vi "DetectExtendCollision.vi"(4 "Ball":T1, 5 "Goal":dbl[](array[numeric]), 6 "Robot in":T2={"id"=0, "function"=enum."Attacker", "x"=0.0, "y"=0.0, "orientation"=0.0, "v_tangent"=0.0, "v_normal"=0.0, "v_ang"=0.0, "kick_x"=0.0, "kick_z"=0.0, "dribble"=FALSE, "Timestamp"=timestamp(0 s since 1904-01-01), "estimatives"={"est_v_tangent"=0.0, "est_v_normal"=0.0, "est_vx"=0.0, "est_vy"=0.0, "Pos Robot Est"=[]}, "dest_x_kick"=0.0, "dest_y_kick"=0.0, "Gap Coord"=[], "States"=enum."GoToTangent", "Path "=[], "Path  Smooth"=[], "Dest"=[]}, 7 "Initial State":dbl[](array[numeric]), 9 "enemy_robots":T2[](array[typedef]), 10 "Point":dbl[](array[numeric]), 11 "our_robots":T2[](array[typedef])) -> (2 "Collision":bool)   [LabVIEW 2017]
uses:
  Core/AI Robot.ctl
  Intel/Functions Enum.ctl
  Intel/AttackerStates.ctl
  PathDests.ctl
  PathDest.ctl
  Core/AI Ball.ctl
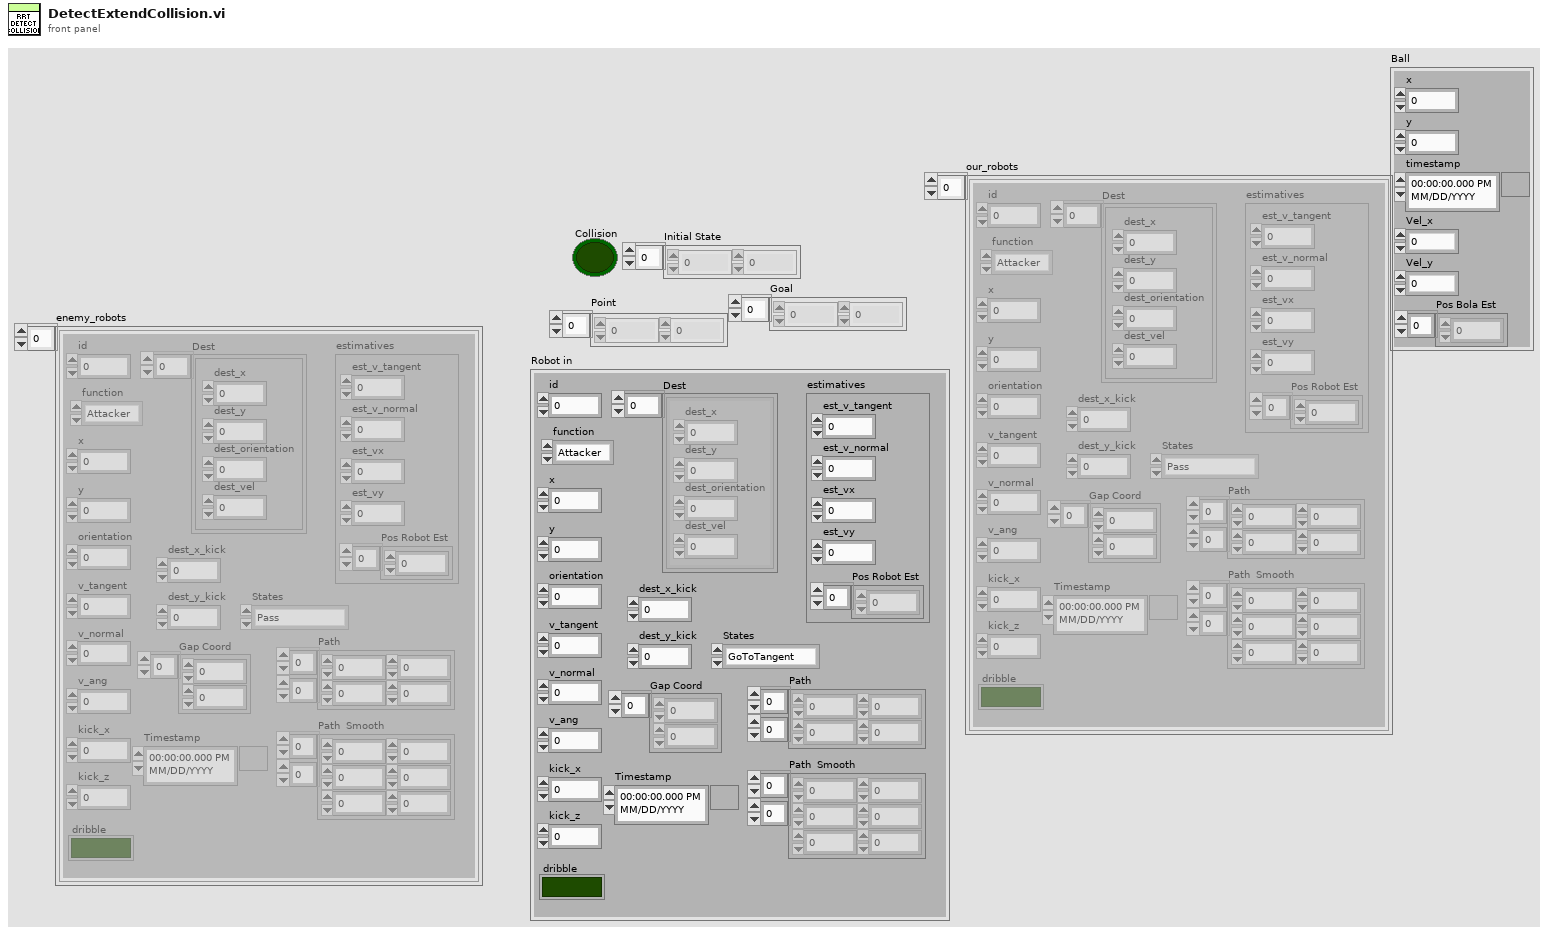
[diagram p1: front panel]
types:
  T1 = typedef "AI Ball.ctl" = cluster{"x":dbl, "y":dbl, "timestamp":timestamp, "Vel_x":dbl, "Vel_y":dbl, "Pos Bola Est":dbl[]}
  T2 = typedef "AI Robot.ctl" = cluster{"id":u32, "function":T3, "x":dbl, "y":dbl, "orientation":dbl, "v_tangent":dbl, "v_normal":dbl, "v_ang":dbl, "kick_x":dbl, "kick_z":dbl, "dribble":bool, "Timestamp":timestamp, "estimatives":cluster{"est_v_tangent":dbl, "est_v_normal":dbl, "est_vx":dbl, "est_vy":dbl, "Pos Robot Est":dbl[]}, "dest_x_kick":dbl, "dest_y_kick":dbl, "Gap Coord":dbl[], "States":T4, "Path ":dbl[][], "Path  Smooth":dbl[][], "Dest":T5}
  T3 = typedef "Functions Enum.ctl" = enum16{"Attacker", "Goalie", "Defender", "Striker", "Goto 0", "Dummy", "Kicker", "ZigZag"}
  T4 = typedef "AttackerStates.ctl" = enum16{"Pass", "GoToTangent", "BallGetting", "GoToKick", ""}
  T5 = typedef "PathDests.ctl" = T6[]
  T6 = typedef "PathDest.ctl" = cluster{"dest_x":dbl, "dest_y":dbl, "dest_orientation":dbl, "dest_vel":dbl}
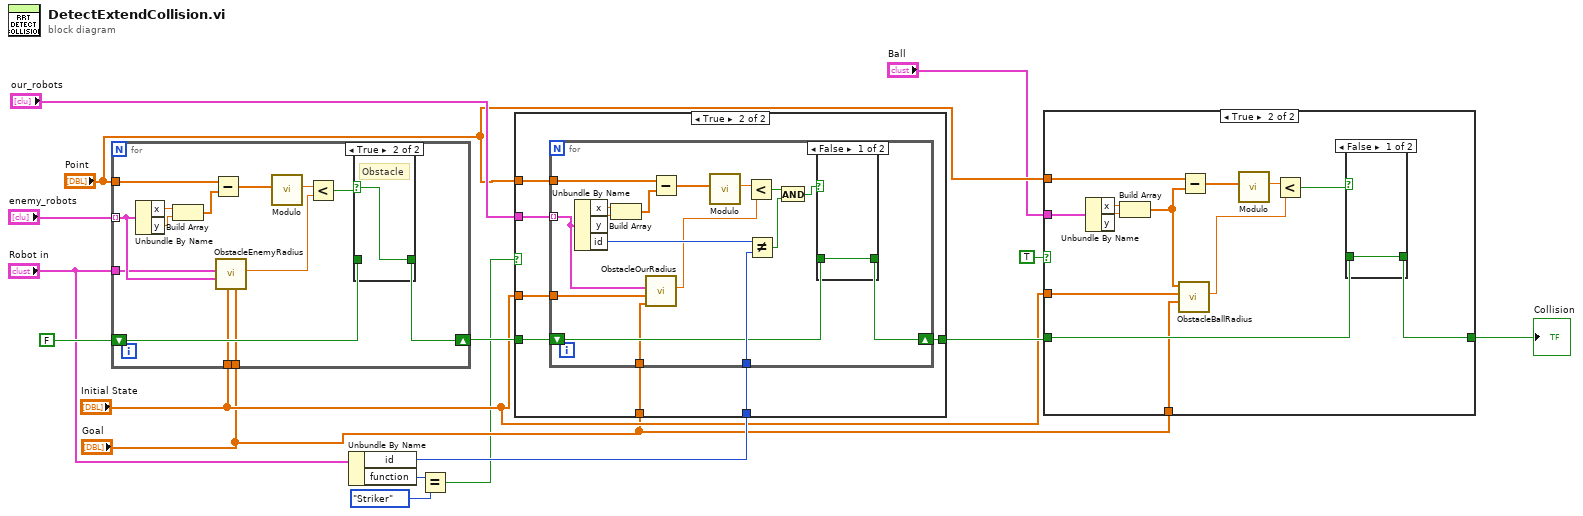
[diagram p0: block diagram]
diagram:
  n1 = for {
    tunnel: "enemy_robots" -> [w20] mode=indexing
    tunnel: "Point" -> [w27]
    shift-right: [w22] -> w11
    shift-left: FALSE -> [w23]
    tunnel: "Robot in" -> [w19]
    tunnel: "Initial State" -> [w18]
    tunnel: "Goal" -> [w17]
    n2 = Unbundle By Name(w20) -> ("x"=w30:dbl, "y"=w29:dbl)
    n3 = Build Array(w30, w29) -> (w28:dbl[])
    n4 = Subtract(x=w27, y=w28) -> (x-y=w26:dbl[])
    n5 = call "ObstacleEnemyRadius.vi"("Goal"=w17, "Initial State"=w18, "Robot enemy"=w20, "Robot in"=w19) -> ("obstacle enemy radius"=w21:dbl)  [unwired: 7 in]
    n6 = call "Modulo.vi"("2D vector"=w26) -> ("Modulo"=w25:dbl)  [unwired: 10 in]
    n7 = Less?(x=w25, y=w21) -> (x < y?=w24:bool)
    n8 = case shown="True" w24 {
      selector: w24 -> [_ w32]
      tunnel: w23 -> [w31 _]
      tunnel: [w31 w32] -> w22
      frame False {
      }
      frame True {
        # "Obstacle"
      }
    }
  }
  n9 = Unbundle By Name("Robot in") -> ("id"=w12:u32, "function"=w3:T3)
  n10 = Equal?(x=w3, y=Functions_Enum."Striker") -> (x = y?=w1:bool)
  n11 = case shown="True" w1 {
    tunnel: w11 -> [w33 w40]
    tunnel: "our_robots" -> [_ w39]
    tunnel: "Point" -> [_ w38]
    tunnel: [w33 w37] -> w8
    tunnel: w12 -> [_ w36]
    tunnel: "Initial State" -> [_ w35]
    tunnel: "Goal" -> [_ w34]
    frame False {
    }
    frame True {
      n12 = for {
        tunnel: w39 -> [w41] mode=indexing
        tunnel: w38 -> [w54]
        shift-right: [w51] -> w37
        shift-left: w40 -> [w45]
        tunnel: w36 -> [w46]
        tunnel: w35 -> [w43]
        tunnel: w34 -> [w42]
        n13 = Unbundle By Name(w41) -> ("x"=w57:dbl, "y"=w56:dbl, "id"=w47:u32)
        n14 = Build Array(w57, w56) -> (w55:dbl[])
        n15 = call "ObstacleOurRadius.vi"("Goal"=w42, "Initial State"=w43, "other robot"=w41) -> ("obstacle enemy radius"=w44:dbl)  [unwired: 8 in]
        n16 = Subtract(x=w54, y=w55) -> (x-y=w53:dbl[])
        n17 = call "Modulo.vi"("2D vector"=w53) -> ("Modulo"=w52:dbl)  [unwired: 10 in]
        n18 = Less?(x=w52, y=w44) -> (x < y?=w50:bool)
        n19 = Not Equal?(x=w47, y=w46) -> (x != y?=w48:bool)
        n20 = And(x=w50, y=w48) -> (x .and. y?=w49:bool)
        n21 = case shown="False" w49 {
          selector: w49 -> [_ w59]
          tunnel: w45 -> [w58 _]
          tunnel: [w58 w59] -> w51
          frame False {
          }
          frame True {
            # "Obstacle"
          }
        }
      }
    }
  }
  n22 = case shown="True" TRUE {
    tunnel: w8 -> [w60 w73]
    tunnel: "Ball" -> [_ w72]
    tunnel: "Point" -> [_ w71]
    tunnel: [w60 w70] -> w10
    tunnel: "Initial State" -> [_ w63]
    tunnel: "Goal" -> [_ w62]
    frame False {
    }
    frame True {
      n23 = Unbundle By Name(w72) -> ("x"=w66:dbl, "y"=w65:dbl)
      n24 = Build Array(w66, w65) -> (w64:dbl[])
      n25 = call "ObstacleBallRadius.vi"("Goal"=w62, "Initial State"=w63, "ball"=w64) -> ("obstacle enemy radius"=w61:dbl)  [unwired: 8 in]
      n26 = Subtract(x=w71, y=w64) -> (x-y=w69:dbl[])
      n27 = call "Modulo.vi"("2D vector"=w69) -> ("Modulo"=w68:dbl)  [unwired: 10 in]
      n28 = Less?(x=w68, y=w61) -> (x < y?=w67:bool)
      n29 = case shown="False" w67 {
        selector: w67 -> [_ w75]
        tunnel: w73 -> [w74 _]
        tunnel: [w74 w75] -> w70
        frame False {
        }
        frame True {
          # "Obstacle"
        }
      }
    }
  }
  "Collision" <- w10
